vi "TestJustCollectCORData.vi"() -> ()   [LabVIEW 2019]
uses:
  enable_disable_enum_typedef.ctl
  MotorController.lvclass
panel:
  out "Error Out":errorcluster
  in  "Serial Port":refnum<visa-resource-name>
  in  "Error In":errorcluster
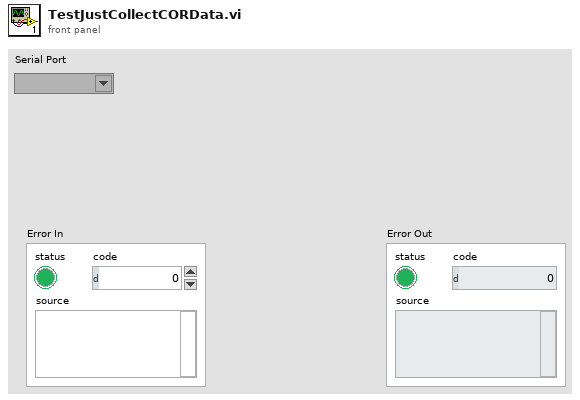
[diagram p1: front panel]
types:
  T1 = typedef "MotorController.lvclass/enable_disable_enum_typedef.ctl" = enum16{"Enable", "Disable"}
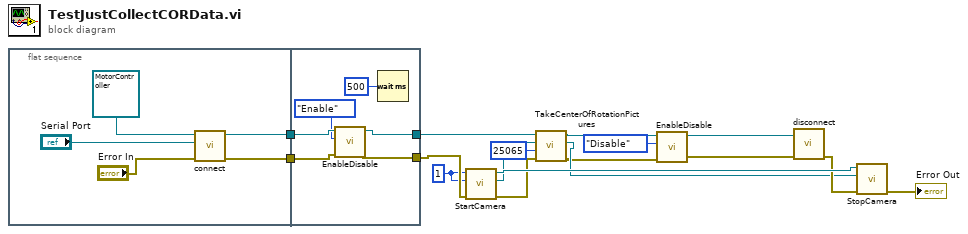
[diagram p0: block diagram]
diagram:
  w14 = u32 1 ("Gain")
  n1 = flat-sequence {
    tunnel: [w20] -> w17
    tunnel: [w19] -> w16
    tunnel: [w27] -> w7
    tunnel: w17 -> [w25]
    tunnel: w16 -> [w24]
    tunnel: [w26] -> w15
    frame #0 {
      n2 = call "connect.vi"("error in (no error)"="Error In", "Serial Port"="Serial Port", "MotorController in"=refnum<class "MotorController.lvclass"> refnum ("MotorController.lvclass")) -> ("error out"=w19:errorcluster, "MotorController out"=w20:refnum<class "MotorController.lvclass">)  [unwired: 7 in]
    }
    frame #1 {
      n3 = call "EnableDisable.vi"("error in (no error)"=w24, "Action"=enable_disable_enum_typedef."Enable", "MotorController in"=w25) -> ("error out"=w26:errorcluster, "MotorController out"=w27:refnum<class "MotorController.lvclass">)  [unwired: 7 in]
      n4 = Wait (ms)(milliseconds to wait=u32 500) -> ()  [unwired: 1 out]
    }
  }
  n5 = call "StartCamera.vi"("Error In"=w15, "ExposureTime_us"=w14, "Gain"=w14) -> ("Error Out"=w3:errorcluster, "TLCamera reference out"=w4:refnum<k24>, "TLCameraSDK reference out"=w13:refnum<k24>)  [unwired: 6 in]
  n6 = call "TakeCenterOfRotationPictures.vi"("Error In"=w3, "Exposure (us)"=u32 25065, "TLCamera reference in"=w4, "MotorController in"=w7) -> ("Error Out"=w1:errorcluster, "TLCamera reference out"=w5:refnum<k24>, "MotorController out"=w6:refnum<class "MotorController.lvclass">)  [unwired: 5 in]
  n7 = call "EnableDisable.vi"("error in (no error)"=w1, "Action"=enable_disable_enum_typedef."Disable", "MotorController in"=w6) -> ("error out"=w9:errorcluster, "MotorController out"=w10:refnum<class "MotorController.lvclass">)  [unwired: 7 in]
  n8 = call "disconnect.vi"("error in (no error)"=w9, "MotorController in"=w10) -> ("error out"=w12:errorcluster)  [unwired: 8 in, 1 out]
  n9 = call "StopCamera.vi"("Error In"=w12, "TLCamera reference"=w5, "TLCameraSDK reference"=w13) -> ("Error Out"=→"Error Out":errorcluster)  [unwired: 8 in]
